vi "GetInputLoopTunnels.vi"(6 "error in":errorcluster, 9 "Loop in":refnum<class "Loop.lvclass">) -> (0 "error out":errorcluster, 3 "Loop out":refnum<class "Loop.lvclass">, 4 "tunnels":refnum<class "LoopTunnel.lvclass">[](array[class]))   [LabVIEW 2014, in "Loop.lvclass"]
uses:
  Loop.lvclass
  LoopTunnel/LoopTunnel.lvclass
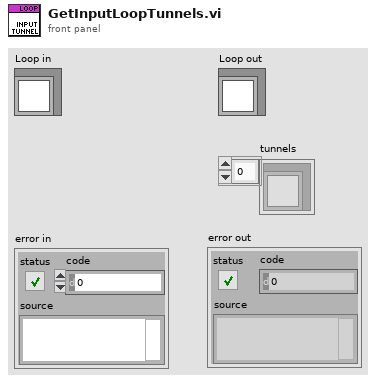
[diagram p1: front panel]
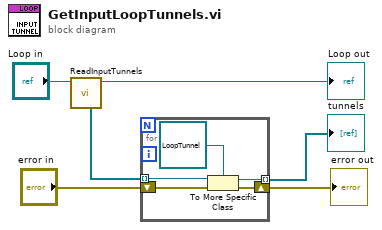
[diagram p0: block diagram]
diagram:
  n1 = call-dynamic "ReadInputTunnels.vi"("Structure in"="Loop in") -> ("Structure out"=→"Loop out":refnum<class "Loop.lvclass">, "tunnels"=w5:refnum<class "Tunnel.lvclass">[])  [unwired: 7 in]
  n2 = for {
    tunnel: w5 -> [w11] mode=indexing
    tunnel: [w9] -> w6 mode=indexing
    shift-right: [w8] -> w1
    shift-left: "error in" -> [w7]
    n3 = To More Specific Class(target class=refnum<class "LoopTunnel.lvclass"> refnum ("LoopTunnel.lvclass"), reference=w11, error in=w7) -> (specific class reference=w9:refnum<class "LoopTunnel.lvclass">, error out=w8:errorcluster)
  }
  "tunnels" <- w6
  "error out" <- w1
